vi "nidaq_Analog_Output.vi"() -> ()   [LabVIEW 2011]
panel:
  in  "stop":bool
  in  "start Solenoide Valve":bool caption="start chromat"
  in  "start chromat":bool
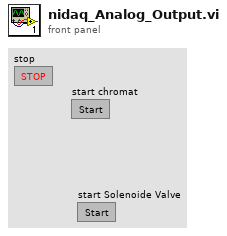
[diagram p1: front panel]
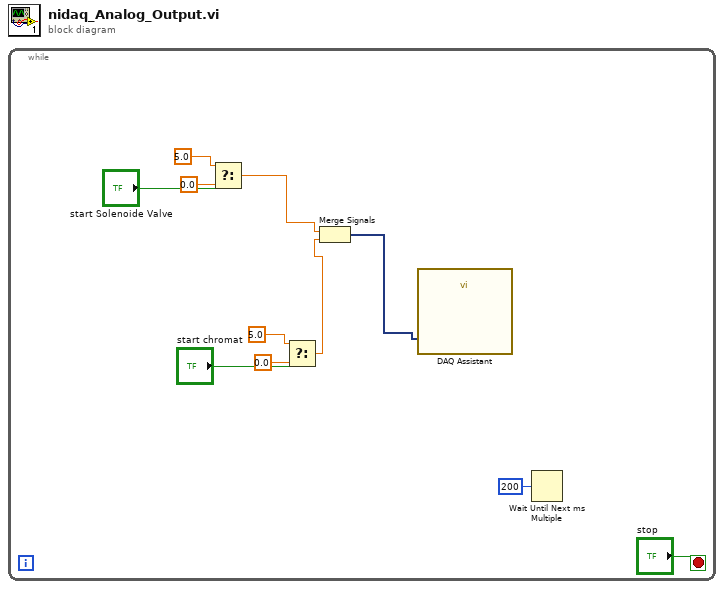
[diagram p0: block diagram]
diagram:
  n1 = while {
    stop <- "stop" stop-if-true
    n2 = Select(t=5.0, s="start Solenoide Valve", f=0.0) -> (s? t:f=w3:dbl)
    n3 = Select(t=5.0, s="start chromat", f=0.0) -> (s? t:f=w7:dbl)
    n4 = Merge Signals(w3, w7) -> (w8:dynamicdata)
    n5 = call "DAQ Assistant"("data"=w8) -> ()  [unwired: 17 in, 2 out]
    n6 = Wait Until Next ms Multiple(millisecond multiple=u32 200) -> ()  [unwired: 1 out]
  }
